vi "IntanConfigure.vi"(8 "error in (no error)":errorcluster, 9 "Record":bool=TRUE, 11 "IntanElectrophysiology.in":refnum<class "IntanElectrophysiology.lvclass">) -> (0 "error out":errorcluster, 3 "IntanElectrophysiology.out":refnum<class "IntanElectrophysiology.lvclass">)   [LabVIEW 2014, in "IntanElectrophysiology.lvclass"]
uses:
  IntanElectrophysiology.lvclass
  IntanElectrophysiology.lvclass/IntanElectrophysiology.ctl
  Electrophysiology/Electrophysiology.lvclass/Electrophysiology.ctl
  AcquireTraces/AcquireTraces.lvclass/AcquireTraces.ctl
  Electrophysiology/Electrophysiology.lvclass
  AcquireTraces/AcquireTraces.lvclass
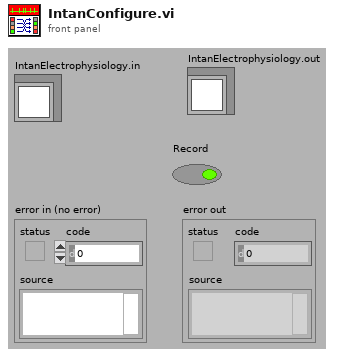
[diagram p1: front panel]
types:
  T1 = cluster{"Channels":string[], "SampClkRate":dbl, "AIDevScalingCoeff":dbl[], "Acq Channel Number":i32[], "Num Preamp Streams":i32, "Chans Per Preamp Stream":i32, "Num Board Channels":i32, "Samples Per Pkt Per Chan":i32}
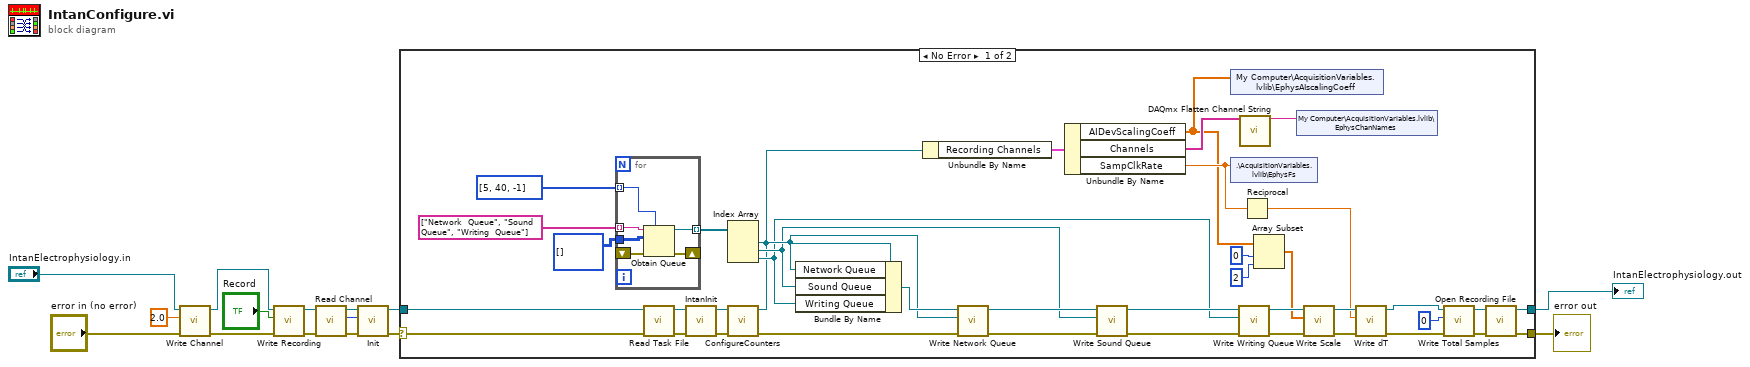
[diagram p0: block diagram]
diagram:
  n1 = call-dynamic "Write Channel.vi"("error in (no error)"="error in (no error)", "Channel"=2.0, "AcquistionObject in"="IntanElectrophysiology.in") -> ("error out"=w8:errorcluster, "AcquistionObject out"=w9:refnum<class "IntanElectrophysiology.lvclass">)  [unwired: 7 in]
  n2 = call-dynamic "Write Recording.vi"("error in (no error)"=w8, "Recording"="Record", "AcquireTraces in"=w9) -> ("error out"=w10:errorcluster, "AcquireTraces out"=w3:refnum<class "IntanElectrophysiology.lvclass">)  [unwired: 7 in]
  n3 = call-dynamic "Read Channel.vi"("error in (no error)"=w10, "AcquistionObject in"=w3) -> ("error out"=w11:errorcluster, "Channel"=w13:i16, "AcquistionObject out"=w12:refnum<class "IntanElectrophysiology.lvclass">)  [unwired: 7 in]
  n4 = call-dynamic "Init.vi"("error in (no error)"=w11, "Channel"=w13, "AcquistionObject in"=w12) -> ("error out"=w1:errorcluster, "AcquistionObject out"=w2:refnum<class "IntanElectrophysiology.lvclass">)  [unwired: 7 in]
  n5 = case shown="No Error" w1 {
    selector: w1 -> [w43 w63]
    tunnel: [w45 w63] -> w6
    tunnel: [w44 w62] -> w5
    tunnel: w2 -> [w26 w62]
    frame No Error {
      n6 = for {
        tunnel: string[] ["Network  Queue", "Sound  Queue", "Writing  Queue"] -> [w61] mode=indexing
        tunnel: i32[][] [] -> [w60]
        tunnel: [w59] -> w53 mode=indexing
        shift-right: [w58] -> _
        shift-left: _ -> [w57]
        tunnel: i32[] [5, 40, -1] -> [w56] mode=indexing
        n7 = Obtain Queue(max queue size (-1, unlimited)=w56, name (unnamed)=w61, element data type=w60, error in (no error)=w57) -> (queue out=w59:refnum<queue>, error out=w58:errorcluster)  [unwired: 1 in, 1 out]
      }
      n8 = call "Read Task File.vi"("error in (no error)"=w43, "IntanElectrophysiology in"=w26) -> ("error out"=w25:errorcluster, "IntanElectrophysiology out"=w22:refnum<class "IntanElectrophysiology.lvclass">)  [unwired: 8 in]
      n9 = call "IntanInit.vi"("error in (no error)"=w25, "IntanElectrophysiology in"=w22) -> ("error out"=w20:errorcluster, "IntanElectrophysiology out"=w21:refnum<class "IntanElectrophysiology.lvclass">)  [unwired: 8 in]
      n10 = Index Array(array=w53) -> (element #1=w41:refnum<queue>, element #2=w39:refnum<queue>, element #3=w37:refnum<queue>)  [unwired: 3 in]
      n11 = call "ConfigureCounters.vi"("error in (no error)"=w20, "IntanElectrophysiology in"=w21) -> ("error out"=w23:errorcluster, "IntanElectrophysiology out"=w24:refnum<class "IntanElectrophysiology.lvclass">)  [unwired: 8 in]
      n12 = Bundle By Name(cluster=w24, "Network Queue"=w41, "Sound Queue"=w39, "Writing Queue"=w37) -> (w42:refnum<class "IntanElectrophysiology.lvclass">)
      n13 = Unbundle By Name(w24) -> ("Recording Channels"=w50:T1)
      n14 = call "Write Network Queue.vi"("error in (no error)"=w23, "Network Queue"=w41, "Electrophysiology in"=w42) -> ("error out"=w35:errorcluster, "Electrophysiology out"=w40:refnum<class "IntanElectrophysiology.lvclass">)  [unwired: 7 in]
      n15 = Unbundle By Name(w50) -> ("AIDevScalingCoeff"=w19:dbl[], "Channels"=w49:string[], "SampClkRate"=w48:dbl)
      n16 = call "Write Sound Queue.vi"("error in (no error)"=w35, "Sound Queue"=w39, "Electrophysiology in"=w40) -> ("error out"=w34:errorcluster, "Electrophysiology out"=w38:refnum<class "IntanElectrophysiology.lvclass">)  [unwired: 7 in]
      n17 = shared-variable "My Computer\\AcquisitionVariables.lvlib\\EphysAIscalingCoeff"(w19) -> ()  [unwired: 1 in, 1 out]
      n18 = shared-variable ".\\AcquisitionVariables.lvlib\\EphysFs"(w48) -> ()  [unwired: 1 in, 1 out]
      n19 = call "Write Writing Queue.vi"("error in (no error)"=w34, "Writing Queue"=w37, "Electrophysiology in"=w38) -> ("error out"=w33:errorcluster, "Electrophysiology out"=w36:refnum<class "IntanElectrophysiology.lvclass">)  [unwired: 7 in]
      n20 = call <vilib>:"DAQmx Flatten Channel String.vi"("names in"=w49) -> ("names out"=w52:string)  [unwired: 13 in, 1 out]
      n21 = Reciprocal(x=w48) -> (1/x=w31:dbl)
      n22 = Array Subset(array=w19, index=0, length=2) -> (w16:dbl[])
      n23 = shared-variable "My Computer\\AcquisitionVariables.lvlib\\EphysChanNames"(w52) -> ()  [unwired: 1 in, 1 out]
      n24 = call-dynamic "Write Scale.vi"("error in (no error)"=w33, "Scale (V/LSB)"=w16, "AcquireTraces in"=w36) -> ("error out"=w46:errorcluster, "AcquireTraces out"=w47:refnum<class "IntanElectrophysiology.lvclass">)  [unwired: 7 in]
      n25 = call-dynamic "Write dT.vi"("error in (no error)"=w46, "dT"=w31, "AcquireTraces in"=w47) -> ("error out"=w28:errorcluster, "AcquireTraces out"=w30:refnum<class "IntanElectrophysiology.lvclass">)  [unwired: 7 in]
      n26 = call "Write Total Samples.vi"("error in (no error)"=w28, "Total Samples"=u64 0, "AcquireTraces in"=w30) -> ("error out"=w27:errorcluster, "AcquireTraces out"=w29:refnum<class "IntanElectrophysiology.lvclass">)  [unwired: 7 in]
      n27 = call-dynamic "Open Recording File.vi"("error in (no error)"=w27, "IntanElectrophysiology in"=w29) -> ("error out"=w45:errorcluster, "IntanElectrophysiology out"=w44:refnum<class "IntanElectrophysiology.lvclass">)  [unwired: 8 in]
    }
    frame Error {
    }
  }
  "error out" <- w6
  "IntanElectrophysiology.out" <- w5
